vi "Find Block Diagram Resource.vi"(11 "Resources":T2) -> (1 "Index":i32, 2 "Found?":bool, 3 "Resource":T1)   [LabVIEW 2017]
uses:
  Find Resource by Type (String).vi
  Resource.ctl
  Resource Array.ctl
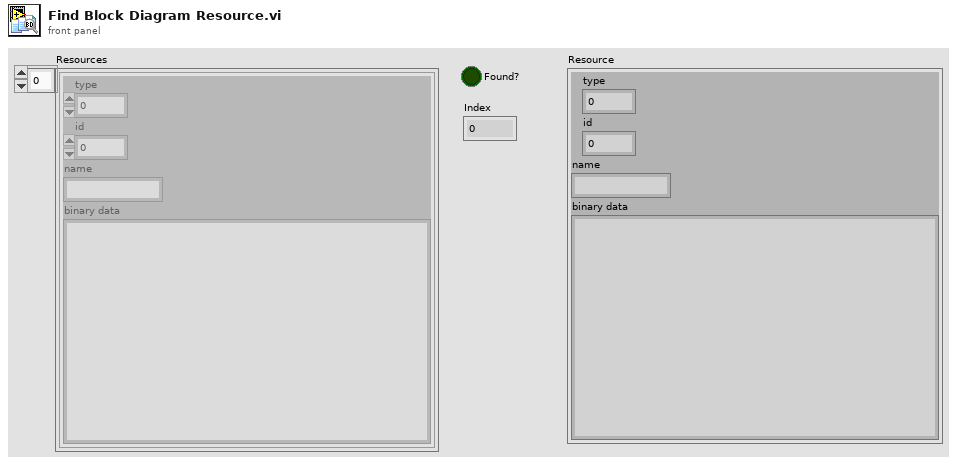
[diagram p1: front panel]
types:
  T1 = typedef "Resource.ctl" = cluster{"type":u32, "id":i32, "name":string, "binary data":string}
  T2 = typedef "Resource Array.ctl" = T1[]
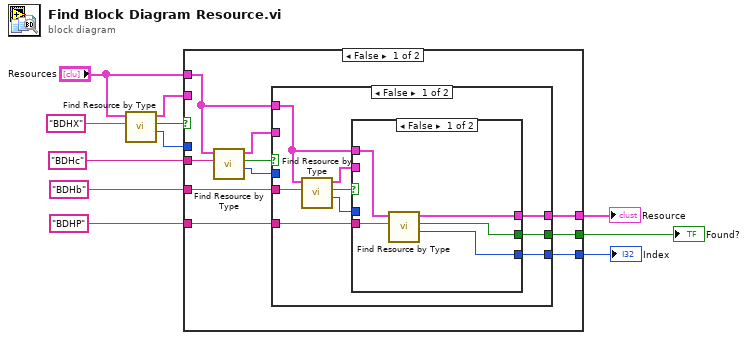
[diagram p0: block diagram]
diagram:
  n1 = call-poly "Find Resource by Type.vi"("Resource Type"="BDHX", "Resources"="Resources") -> ("Index"=w1:i32, "Found?"=w10:bool, "Resource"=w2:T1)  [unwired: 7 in]
  n2 = case shown="False" w10 {
    selector: w10 -> [_ w43]
    tunnel: "BDHc" -> [w21 _]
    tunnel: "BDHb" -> [w19 _]
    tunnel: "Resources" -> [w18 _]
    tunnel: "BDHP" -> [w17 _]
    tunnel: [w16 w44] -> w4
    tunnel: [w15 w43] -> w3
    tunnel: [w14 w42] -> w5
    tunnel: w2 -> [_ w44]
    tunnel: w1 -> [_ w42]
    frame False {
      n3 = call-poly "Find Resource by Type.vi"("Resource Type"=w21, "Resources"=w18) -> ("Index"=w12:i32, "Found?"=w20:bool, "Resource"=w13:T1)  [unwired: 7 in]
      n4 = case shown="False" w20 {
        selector: w20 -> [_ w40]
        tunnel: w19 -> [w30 _]
        tunnel: w18 -> [w28 _]
        tunnel: w17 -> [w27 _]
        tunnel: [w26 w41] -> w16
        tunnel: [w25 w40] -> w15
        tunnel: [w24 w39] -> w14
        tunnel: w13 -> [_ w41]
        tunnel: w12 -> [_ w39]
        frame False {
          n5 = call-poly "Find Resource by Type.vi"("Resource Type"=w30, "Resources"=w28) -> ("Index"=w22:i32, "Found?"=w29:bool, "Resource"=w23:T1)  [unwired: 7 in]
          n6 = case shown="False" w29 {
            selector: w29 -> [_ w36]
            tunnel: w28 -> [w35 _]
            tunnel: w27 -> [w34 _]
            tunnel: [w33 w38] -> w26
            tunnel: [w32 w36] -> w25
            tunnel: [w31 w37] -> w24
            tunnel: w23 -> [_ w38]
            tunnel: w22 -> [_ w37]
            frame False {
              n7 = call-poly "Find Resource by Type.vi"("Resource Type"=w34, "Resources"=w35) -> ("Index"=w31:i32, "Found?"=w32:bool, "Resource"=w33:T1)  [unwired: 7 in]
            }
            frame True {
            }
          }
        }
        frame True {
        }
      }
    }
    frame True {
    }
  }
  "Resource" <- w4
  "Found?" <- w3
  "Index" <- w5
